vi "initialize.vi"(0 "HGF_FGV_Visitor":refnum<class "HGF_FGV_Visitor.lvclass">, 3 "initializationData":variant, 5 "error in (no error)":errorcluster, 7 "binaryString":string, 8 "I8 Array":i8[](array[numeric]), 9 "prependSize? (T)":bool, 11 "byteOrder (0:big-endian, network order)":T1(ring)) -> (14 "dup HGF_FGV_Visitor":refnum<class "HGF_FGV_Visitor.lvclass">, 17 "found?":bool, 19 "error out":errorcluster)   [LabVIEW 2012, in "HGF_FGV.lvlib" / "HGF_FGV_Visitor.lvclass"]
doc: "This is a dynamic dispatch VI to be implemented by child classes to initialize their attributes.\n\n<B>Attention:</B> Support for Variant for initialization data only."
uses:
  HGF_FGV_Visitor.lvclass
  HGF_Visitor/HGF_Visitor.lvclass
  HGF_FGV_Action/HGF_FGV_Action.lvclass
  HGF_FGV_Visitor.lvclass/HGF_FGV_Visitor.ctl
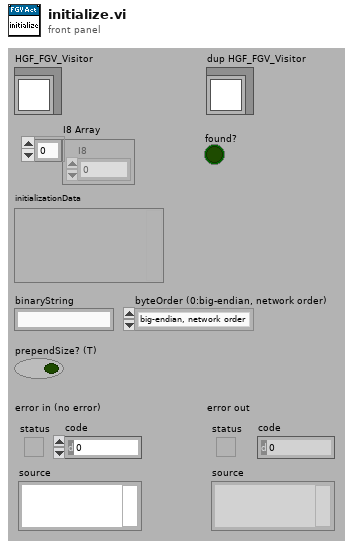
[diagram p1: front panel]
types:
  T1 = enum16{"big-endian, network order", "native, host order", "little-endian"}
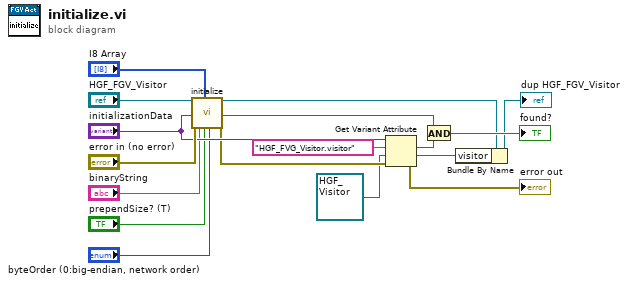
[diagram p0: block diagram]
diagram:
  n1 = call-parent "initialize.vi"("HGF_Factory"="HGF_FGV_Visitor", "initializationData"="initializationData", "error in (no error)"="error in (no error)", "binaryString"="binaryString", "I8 Array"="I8 Array", "prependSize? (T)"="prependSize? (T)", "byteOrder (0:big-endian, network order)"="byteOrder (0:big-endian, network order)") -> ("dup HGF_Factory"=w6:refnum<class "HGF_FGV_Visitor.lvclass">, "found?"=w10:bool, "error out"=w12:errorcluster)  [unwired: 1 in, 9 out]
  n2 = Get Variant Attribute(Variant="initializationData", name="HGF_FVG_Visitor.visitor", default value (empty Variant)=refnum<class "HGF_Visitor.lvclass"> refnum ("HGF_Visitor.lvclass"), error in=w12) -> (found=w9:bool, value=w4:refnum<class "HGF_Visitor.lvclass">, error out=→"error out":errorcluster)  [unwired: 1 out]
  n3 = And(x=w10, y=w9) -> (x .and. y?=→"found?":bool)
  n4 = Bundle By Name(cluster=w6, "visitor"=w4) -> (→"dup HGF_FGV_Visitor":refnum<class "HGF_FGV_Visitor.lvclass">)
